vi "get result string.vi"(11 "input_test_results":bool[](array[boolean])) -> (3 "results string":string[](array[string]))   [LabVIEW 2011]
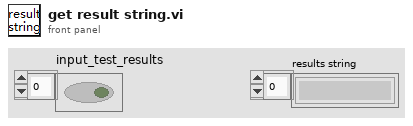
[diagram p1: front panel]
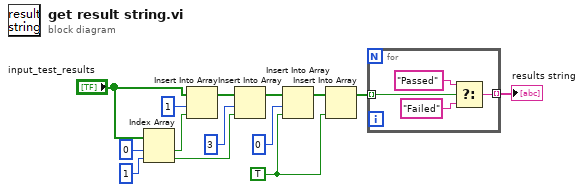
[diagram p0: block diagram]
diagram:
  w4 = TRUE ("新元素/子数组")
  n1 = Index Array(array="input_test_results", index #1=0 ("索引"), index #2=1 ("索引")) -> (element #1=w12:bool, element #2=w9:bool)
  n2 = Insert Into Array(array="input_test_results", index=1 ("索引"), new element=w12) -> (w10:bool[])
  n3 = Insert Into Array(array=w10, index=3 ("索引"), new element=w9) -> (w7:bool[])
  n4 = Insert Into Array(array=w7, index=0 ("索引"), new element=w4) -> (w5:bool[])
  n5 = Insert Into Array(array=w5, new element=w4) -> (w2:bool[])  [unwired: 1 in]
  n6 = for {
    tunnel: w2 -> [w18] mode=indexing
    tunnel: [w15] -> w1 mode=indexing
    n7 = Select(t="Passed", s=w18, f="Failed") -> (s? t:f=w15:string)
  }
  "results string" <- w1
